vi "Source Output Enable.vi"(7 "Output (Off)":bool, 8 "error in (no error)":errorcluster, 9 "Channel (Channel A)":T1, 10 "Node In":string, 11 "VISA resource name":refnum<visa-resource-name>) -> (0 "error out":errorcluster, 2 "Node Out":string, 3 "VISA resource name out":refnum<visa-resource-name>, 4 "Command String":string)   [LabVIEW 2025, in "MySMU.lvlib"]
doc: "This VI turns the SMU output on or off.\n\n<b>Functions and Attributes Used</b>\nsmuX.source.output"
uses:
  MySMU.lvlib
  Channel.ctl
  GlobalVariables.vi
panel:
  # "(c) 2008 Keithley Instruments, Inc.  ALL RIGHTS RESERVED."
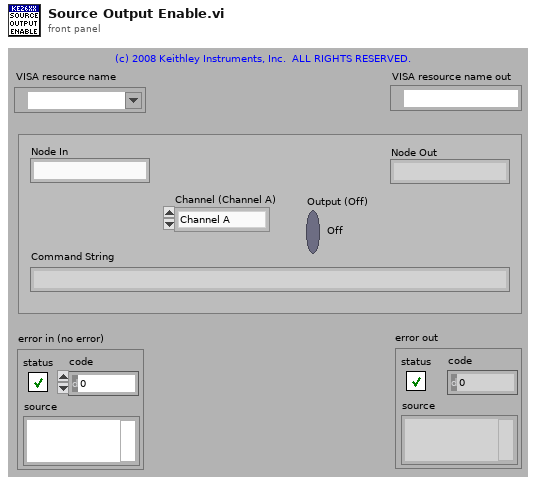
[diagram p1: front panel]
types:
  T1 = typedef "MySMU.lvlib/Channel.ctl" = enum32{"Channel A", "Channel B"}
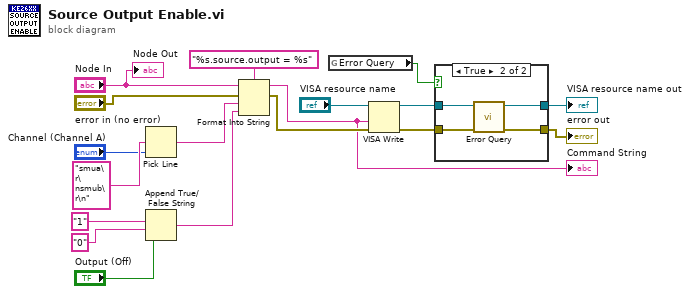
[diagram p0: block diagram]
diagram:
  n1 = Pick Line(multi-line string="smua\r\nsmub\r\n" ("options"), line index="Channel (Channel A)") -> (output string=w6:string)  [unwired: 1 out]
  n2 = Append True/False String(1:"Output (Off)", 2:"0" ("false string"), 3:"1" ("true string")) -> (0:w5:string)  [unwired: 1 out]
  n3 = Format Into String(format string="%s.source.output = %s", initial string="Node In", error in="error in (no error)", w6, w5) -> (resulting string=w1:string, error out=w2:errorcluster)
  "Command String" <- w1
  n4 = global read "GlobalVariables.vi" "Error Query"() -> (w13:bool)
  n5 = VISA Write(VISA resource name="VISA resource name", write buffer=w1, error in (no error)=w2) -> (VISA resource name out=w12:refnum<visa-resource-name>, error out=w11:errorcluster)  [unwired: 1 out]
  n6 = case shown="True" w13 {
    tunnel: w12 -> [w20 w24]
    tunnel: w11 -> [w19 w23]
    tunnel: [w20 w22] -> w10
    tunnel: [w19 w21] -> w9
    frame False {
    }
    frame True {
      n7 = call "Error Query.vi"("error in (no error)"=w23, "VISA resource name"=w24) -> ("error out"=w21:errorcluster, "VISA resource name out"=w22:refnum<visa-resource-name>)  [unwired: 8 out]
    }
  }
  "VISA resource name out" <- w10
  "error out" <- w9
  "Node Out" <- "Node In"
